vi "Decompose KVPs.vi"(9 "Name (empty: value name)":string, 11 "value":variant) -> (1 "Values":variant[](array[variant]), 3 "Keys":string[](array[string]))   [LabVIEW 2013, in "CfgManager.lvlib" / "ConfigManager.lvclass"]
uses:
  ConfigManager.lvclass
  <vilib>/LabVIEW Open Source/Data Manipulation/TypeDescriptor/TypeDescriptor_GetName.vi
  <vilib>/LabVIEW Open Source/Data Manipulation/TypeDescriptor/TypeDescriptor_GetPString.vi
  <vilib>/LabVIEW Open Source/Data Manipulation/TypeDescriptor/TypeDescriptor_SetName.vi
  <vilib>/LabVIEW Open Source/Data Manipulation/Variant/OpenVariant.lvlib
  <vilib>/Utility/VariantDataType/VariantType.lvlib
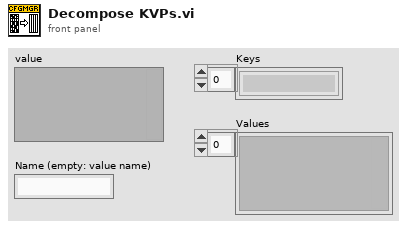
[diagram p1: front panel]
types:
  T1 = typedef "VariantType.lvlib/Type.ctl" = enum8{"Invalid Type", "Void", "I8", "I16", "I32", "I64", "U8", "U16", "U32", "U64", "Single Float", "Double Float", "Extended Float", "Single Complex", "Double Complex", "Extended Complex", "Enum U8", "Enum U16", "Enum U32", "Enum U64", "Single Float With Unit", "Double Float With Unit", "Extended Float With Unit", "Single Complex with Unit", "Double Complex with Unit", "Extended Complex with Unit", "Boolean", "String", "Path", "Picture", "Tag", "Array", "Cluster", "Variant", "LV Variant", "Waveform", "Timestamp", "Digital Waveform", "Digital Data", "ExpressData", "Refnum", "External Data", "VI", "Poly VI", "LabVIEW Class Instance", "Fixed Point"}
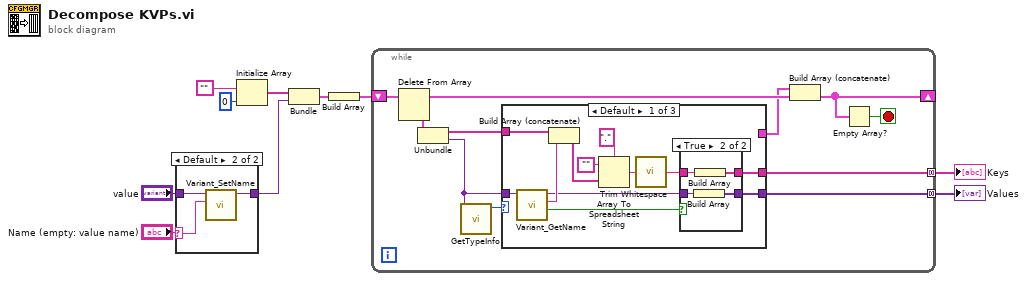
[diagram p0: block diagram]
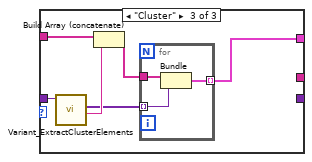
[diagram p4: hidden frame]
diagram:
  n1 = case shown="Default" "Name (empty: value name)" {
    selector: "Name (empty: value name)" -> [_ w13]
    tunnel: "value" -> [w11 w14]
    tunnel: [w11 w12] -> w3
    frame "" {
    }
    frame Default {
      n2 = call <vilib>:"Variant_SetName.vi"("Name"=w13, "Variant"=w14) -> ("Named Variant"=w12:variant)  [unwired: 9 in]
    }
  }
  n3 = Initialize Array("", 0 ("dimension size")) -> (w8:string[])
  n4 = Bundle(w8, "Named Variant"=w3) -> (w4:cluster{string[], "Named Variant":variant})  [unwired: 1 in]
  n5 = Build Array(w4) -> (w5:cluster{string[], "Named Variant":variant}[])
  n6 = while {
    shift-right: [w21] -> _
    shift-left: w5 -> [w24]
    tunnel: [w18] -> w10 mode=concatenating
    tunnel: [w16] -> w9 mode=concatenating
    stop <- w22 stop-if-true
    n7 = Delete From Array(array=w24) -> (deleted portion=w20:cluster{string[], "Named Variant":variant}, array with subset deleted=w23:cluster{string[], "Named Variant":variant}[])  [unwired: 2 in]
    n8 = Unbundle(w20) -> (w17:string[], "Named Variant"=w19:variant)
    n9 = call <vilib>:"GetTypeInfo.vi"("Variant"=w19) -> ("Type Enum"=w25:T1)  [unwired: 6 in, 4 out]
    n10 = case shown="Default" w25 {
      tunnel: w19 -> [w36 _ w47]
      tunnel: [w37 _ _] -> w18
      tunnel: w17 -> [w35 _ w46]
      tunnel: [w28 _ _] -> w16
      tunnel: [_ _ w43] -> w15
      frame Default {
        n11 = call <vilib>:"Variant_GetName.vi"("Variant"=w36) -> ("found"=w26:bool, "Name"=w34:string, "Variant dup"=w27:variant)  [unwired: 8 in]
        n12 = Build Array (concatenate)(w35, w34) -> (w33:string[])
        n13 = Array To Spreadsheet String(delimiter (Tab)=".", array=w33, 3:"") -> (spreadsheet string=w32:string)
        n14 = call <vilib>:"Trim Whitespace.vi"("string"=w32) -> ("trimmed string"=w29:string)  [unwired: 1 in]
        n15 = case shown="True" w26 {
          tunnel: [_ w41] -> w37
          tunnel: w29 -> [_ w40]
          tunnel: [_ w39] -> w28
          tunnel: w27 -> [_ w38]
          frame False {
          }
          frame True {
            n16 = Build Array(w38) -> (w41:variant[])
            n17 = Build Array(w40) -> (w39:string[])
          }
        }
      }
      frame "Invalid Type", "Void" {
      }
      frame "Cluster" {
        n18 = call <vilib>:"Variant_ExtractClusterElements.vi"("Cluster"=w47) -> ("name"=w45:string, "Elements"=w44:variant[])  [unwired: 8 in, 1 out]
        n19 = Build Array (concatenate)(w46, w45) -> (w42:string[])
        n20 = for {
          tunnel: w44 -> [w50] mode=indexing
          tunnel: [w49] -> w43 mode=indexing
          tunnel: w42 -> [w48]
          n21 = Bundle(w48, "Variant"=w50) -> (w49:cluster{string[], "Variant":variant})  [unwired: 1 in]
        }
      }
    }
    n22 = Build Array (concatenate)(w15, w23) -> (w21:cluster{string[], "Named Variant":variant}[])
    n23 = Empty Array?(array=w21) -> (empty?=w22:bool)
  }
  "Values" <- w10
  "Keys" <- w9
